vi "Auto Reset List Box.vi"(8 "error in (no error)":errorcluster, 11 "MulticolumnListbox in":refnum<vi>) -> (0 "error out":errorcluster)   [LabVIEW 2017]
uses:
  <vilib>/Utility/miscctls.llb/LVRowAndColumnTypeDef.ctl
  <vilib>/Utility/miscctls.llb/LVRowAndColumnUnsignedTypeDef.ctl
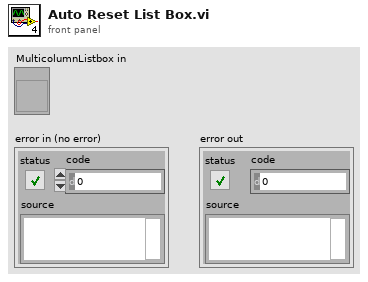
[diagram p1: front panel]
types:
  T1 = typedef "LVRowAndColumnUnsignedTypeDef.ctl" = cluster{"Row":u32, "Column":u32}
  T2 = typedef "LVRowAndColumnTypeDef.ctl" = cluster{"Row":i32, "Column":i32}
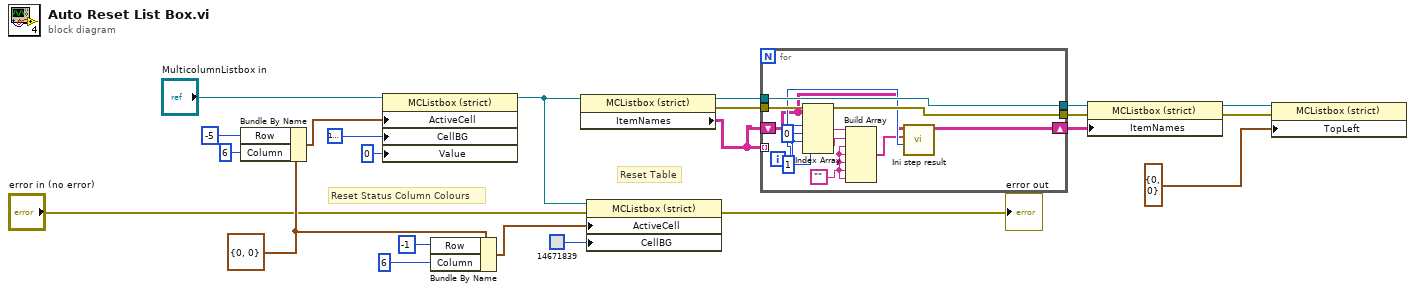
[diagram p0: block diagram]
diagram:
  w20 = T2 {"Row"=0, "Column"=0} ("Active Cell:Active Cell")
  # "Reset Table"
  # "Reset Status Column Colours"
  n1 = Bundle By Name(cluster=w20, "Row"=-5, "Column"=6) -> (w11:T2)
  n2 = property class="MCListbox (strict)"(reference="MulticolumnListbox in", "ActiveCell"=w11, "CellBG"=u32 16777226, "Value"=0) -> (reference out=w16:refnum<vi>)  [unwired: 1 in, 1 out]
  n3 = Bundle By Name(cluster=w20, "Row"=-1, "Column"=6) -> (w23:T2)
  n4 = property class="MCListbox (strict)"(reference=w16) -> (reference out=w6:refnum<vi>, error out=w9:errorcluster, "ItemNames"=w4:string[][])  [unwired: 1 in]
  n5 = property class="MCListbox (strict)"(reference=w16, error in="error in (no error)", "ActiveCell"=w23, "CellBG"=u32 14671839) -> (error out=→"error out":errorcluster)  [unwired: 1 out]
  n6 = for {
    tunnel: w4 -> [_] mode=indexing
    tunnel: w9 -> [w34]
    tunnel: [w34] -> w8
    tunnel: w6 -> [w32]
    tunnel: [w32] -> w5
    shift-right: [w33] -> w7
    shift-left: w4 -> [w24]
    i -> [w31]
    w28 = ""
    n7 = Index Array(array=w24, index (row) #1=w31, index (col) #1=0 ("disabled index (col)"), index (row) #2=w31, index (col) #2=1 ("disabled index (col)")) -> (element #1=w30:string, element #2=w29:string)
    n8 = Build Array(w30, w29, w28, w28, w28, w28, w28) -> (w27:string[])
    n9 = call "Ini step result.vi"("index (row)"=w31, "new element/subarray"=w27, "Out Data"=w24) -> ("output array"=w33:string[][])  [unwired: 8 in]
  }
  n10 = property class="MCListbox (strict)"(reference=w5, error in=w8, "ItemNames"=w7) -> (reference out=w3:refnum<vi>, error out=w2:errorcluster)
  n11 = property class="MCListbox (strict)"(reference=w3, error in=w2, "TopLeft"=T1 {"Row"=0, "Column"=0} ("Top Left Visible Cell")) -> ()  [unwired: 2 out]
